vi "LaunchApp.vi"() -> ()   [LabVIEW 2020, in "CameraTestingLauncher.lvlib"]
uses:
  CameraTestingLauncher.lvlib
  CameraTestingUI/CameraTestingUI/CameraTestingUI.lvclass
  E:/GitHub/Evaluation_Test/Labview/src/CameraTestingApp/ICameraTestingUI/ICameraTestingUI/ICameraTestingUI.lvclass
  ICameraTesting/ICameraTesting/TypeDef/CameraInfo.ctl
  Camera/ICamera/ICamera/ICamera.lvclass
  CameraTesting/CameraTesting/CameraTesting.lvclass
  Camera/CameraI2COUSB/Camera/Camera.lvclass
  E:/GitHub/Evaluation_Test/Labview/src/Camera/ICamera/ICamera/ICamera.lvclass
  Camera/CameraUSB/Camera/Camera.lvclass
  8969cb9a-2b55-45df-ae2b-8a6d22d76d82.vi
  ICameraTesting/ICameraTesting/ICameraTesting.lvclass
panel:
  in  "StartProg":bool
  out "error out":errorcluster
  in  "Camera Type":enum32{"I2COUSB", "USB", "Ethernet", "IMAQ"}(tab)
  in  "I2COOUSBParams":T1
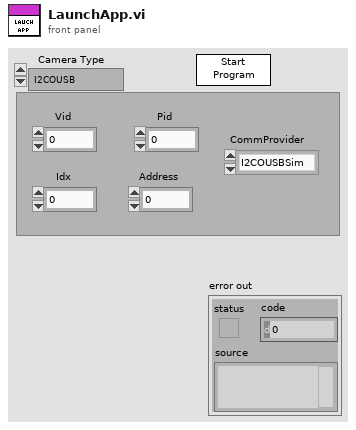
[diagram p1: front panel]
types:
  T1 = cluster{"Vid":u32, "Pid":u32, "Idx":u32, "Address":u32, "CommProvider":enum16{"I2COUSBSim", "ProdType_1", "ProdType_2", "Prod_Type_i", "ProdType_n"}}
  T2 = typedef "ICameraTesting.lvlib/ICameraTesting.lvclass/CameraInfo.ctl" = cluster{"ICamera ":refnum<class "ICamera.lvclass">, "Connection String":string}
  T3 = enum16{"I2COUSBSim", "ProdType_1", "ProdType_2", "Prod_Type_i", "ProdType_n"}
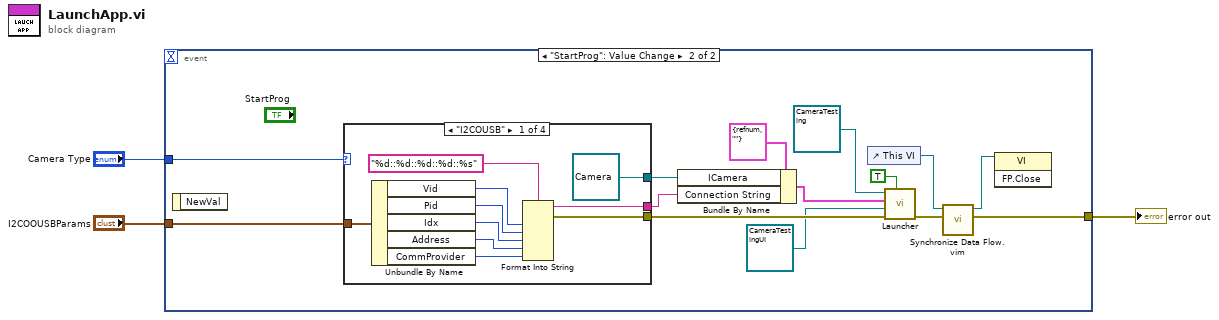
[diagram p0: block diagram]
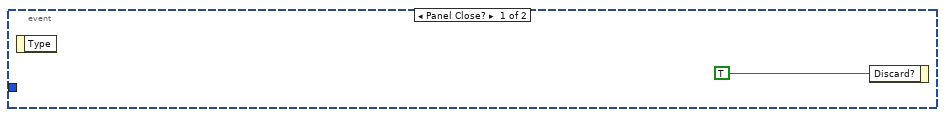
[diagram p2: hidden frame]
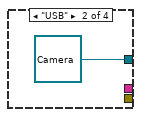
[diagram p3: hidden frame]
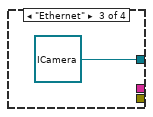
[diagram p4: hidden frame]
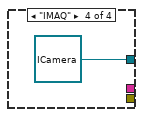
[diagram p5: hidden frame]
diagram:
  n1 = event shown="[1] \"StartProg\": Value Change" {
    selector: _ -> [_ _]
    dyn-events: _ -> [_ _]
    timeout: _ -> [_ _]
    tunnel: "I2COOUSBParams" -> [_ w15]
    tunnel: "Camera Type" -> [_ w14]
    tunnel: [_ w13] -> w1
    event Panel Close? {
      n2 = event-data() -> ()  [unwired: 1 in, 1 out]
      n3 = event-data("Discard?"=TRUE) -> ()  [unwired: 1 in, 1 out]
    }
    event "StartProg": Value Change {
      n4 = event-data() -> ()  [unwired: 1 in, 1 out]
      n5 = case shown="\"I2COUSB\"" w14 {
        tunnel: w15 -> [w27 _ _ _]
        tunnel: [refnum<class "Camera.lvclass"> refnum ("CameraDemo in") refnum<class "Camera.lvclass"> refnum ("CameraUSB.lvlib:Camera.lvclass") refnum<class "ICamera.lvclass"> refnum ("ICamera.lvlib:ICamera.lvclass") refnum<class "ICamera.lvclass"> refnum ("ICamera.lvlib:ICamera.lvclass")] -> w8
        tunnel: [w20 _ _ _] -> w7
        tunnel: [w19 _ _ _] -> w11
        frame "I2COUSB" {
          n6 = Unbundle By Name(w27) -> ("Vid"=w26:u32, "Pid"=w25:u32, "Idx"=w24:u32, "Address"=w23:u32, "CommProvider"=w22:T3)
          n7 = Format Into String(format string="%d::%d::%d::%d::%s", w26, w25, w24, w23, w22) -> (resulting string=w20:string, error out=w19:errorcluster)  [unwired: 2 in]
        }
        frame "USB" {
        }
        frame "Ethernet" {
        }
        frame "IMAQ" {
        }
      }
      n8 = Bundle By Name(cluster=T2 {"ICamera "=refnum, "Connection String"=""} ("CameraInfo"), "ICamera"=w8, "Connection String"=w7) -> (w6:T2)
      n9 = control-ref of="This VI"() -> (w17:refnum<vi>)
      n10 = call-dynamic "Launcher.vi"("Open FP?"=TRUE, "error in (no error)"=w11, "ICameraTestingUI"=refnum<class "CameraTestingUI.lvclass"> refnum ("CameraTestingUI.lvlib:CameraTestingUI.lvclass"), "CameraInfo"=w6, "CameraTesting"=refnum<class "CameraTesting.lvclass"> refnum ("CameraTesting.lvlib:CameraTesting.lvclass")) -> ("error out"=w16:errorcluster)  [unwired: 5 in, 1 out]
      n11 = call "Synchronize Data Flow.vim"("input 2"=w16, "input 1"=w17) -> ("output 2"=w13:errorcluster, "output 1"=w18:refnum<vi>)  [unwired: 2 in, 2 out]
      n12 = invoke class="VI" method="FP.Close"(reference=w18) -> ()  [unwired: 2 in, 3 out]
    }
  }
  "error out" <- w1
